vi "Write Attribute Pointer Flag.vi"(10 "Attribute Pointer?":bool[](array[boolean]), 11 "Conditional Dialog in":refnum<class "Conditional Dialog.lvclass">) -> (3 "Conditional Dialog out":refnum<class "Conditional Dialog.lvclass">)   [LabVIEW 2017, in "Conditional Dialog.lvclass"]
uses:
  <vilib>/gpm_packages/@cs/Test-executive-builder/Source/Test Executive Builder Dialogs/Edit Conditional Dialog/Conditional Dialog.lvclass
  <vilib>/gpm_packages/@cs/Test-executive-builder/Source/Test Executive Builder Dialogs/Edit Conditional Dialog/Conditional Dialog.lvclass/Conditional Dialog.ctl
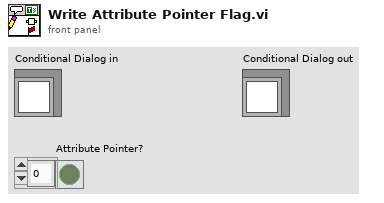
[diagram p1: front panel]
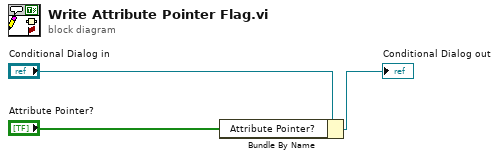
[diagram p0: block diagram]
diagram:
  n1 = Bundle By Name(cluster="Conditional Dialog in", "Attribute Pointer?"="Attribute Pointer?") -> (→"Conditional Dialog out":refnum<class "Conditional Dialog.lvclass">)
